vi "SVT Fractional-octave Analysis (1 Ch).vi"(0 "scaled signal [EU]":waveform(dbl)={"t0"=timestamp(0 s since 1904-01-01), "dt"=1.953125e-05, "Y"=[]}, 1 "restart averaging (F)":bool, 2 "reset filter (F)":bool, 5 "frequency range [Hz]":T9={"low frequency"=125.0, "high frequency"=8000.0} {"high frequency" min=0.001 format="%.2f"; "low frequency" min=0.001 format="%.2f"}, 7 "bandwidth":T2(ring)=enum."1/12 octave", 9 "dB On (T)":bool=TRUE, 11 "error in (no error)":errorcluster, 12 "averaging type":T7(ring), 13 "exp avg settings":T1={" mode"=enum."Fast", "time constant [ms]"=125.0} {"time constant [ms]" format="%.2f"}, 14 "equal confidence level [dB]":dbl=125.0 format="%.2f") -> (3 "filter settled":bool, 4 "octave spectrum":T8 {"band power" format="%.2f"; "nominal frequencies [Hz]" format="%.2f"}, 6 "unit label":string, 8 "total band power":dbl format="%.2f", 10 "octave info":T3={"standard"=enum."ANSI S1.11", "bandwidth"=enum."1 octave", "low band"=0, "high band"=0, "weighting filter"=0, "dB reference"=0.0, "dB On"=FALSE, "unit label"="", "channel name"="", "description"="", "engineering units"=1, "custom label"="", "spectrum type"=enum."magnitude", "spectral density"=FALSE, "filters settled"=FALSE} {"engineering units" items=["custom..."=0, "V"=1, "A"=21, "C"=30, "pC"=31, "s"=32, "-"=29, "Pa"=2, "N"=20, "g"=3, "m/s^2"=4, "m/s"=5, "m"=6, "mm/s"=12, "mm"=13, "micron/s"=14, "micron"=15, "in/s^2"=7, "in/s"=8, "in"=9, "mil/s"=10, "mil"=11, "rad/s^2"=16, "rad/s"=17, "rad"=18, "deg/s^2"=26, "deg/s"=27, "deg"=28, "RPM"=22, "cycle/s^2"=23, "Hz"=24, "cycle"=25, "strain"=19]; "dB reference" format="%.2e"; "weighting filter" items=["Linear", "A-weighting", "B-weighting", "C-weighting", "ITU-R 468-4", "Dolby", "CCITT", "C-message", "Wb", "Wc", "Wd", "We", "Wf", "Wh", "Wj", "Wk", "Wm", "AES17 20 kHz lowpass", "AES17 40 kHz lowpass", "AES17 20 kHz highpass", "AES17 40 kHz highpass"]}, 15 "error out":errorcluster)   [LabVIEW 2017, in "SoundVib_Octave.lvlib"]
doc: "LabVIEW no longer supports this VI. The SVT Fractional-octave Analysis VI is available for compatibility with previous versions of the LabVIEW Sound and Vibration Toolkit. This version of the SVT Fractional-octave Analysis VI performs a fractional-octave analysis on <B>scaled signal [EU]</B> in accordance with the IEC 1260 standard. This standard has been superseded by the new IEC 61260 standard. If you want to ensure compliance with the latter standard, use the SVT Fractional-octave Analysis VI, located on the Octave Analysis palette instead. You can use this polymorphic VI to perform fractional-octave analysis on a single channel or on N channels. The data type you wire to the <B>scaled signal [EU]</B> input determines the polymorphic instance to use."
uses:
  <vilib>/addons/Sound and Vibration/svt_Octave/SoundVib_Octave.lvlib
  <vilib>/addons/_NISVFA/_Shared subVIs/Controls/svc_Octave Info.ctl
  <vilib>/addons/_NISVFA/_Shared subVIs/Controls/svc_Octave Standard.ctl
  <vilib>/addons/_NISVFA/_Shared subVIs/Controls/svc_Weighting Filter Text Ring.ctl
  <vilib>/addons/_NISVFA/_Shared subVIs/Controls/svc_Engineering Units Text Ring.ctl
  <vilib>/addons/Sound and Vibration/svt_Octave_2014 standard/SoundVib_Octave_2014 standard.lvlib
panel:
  out "# samples to settle":u64
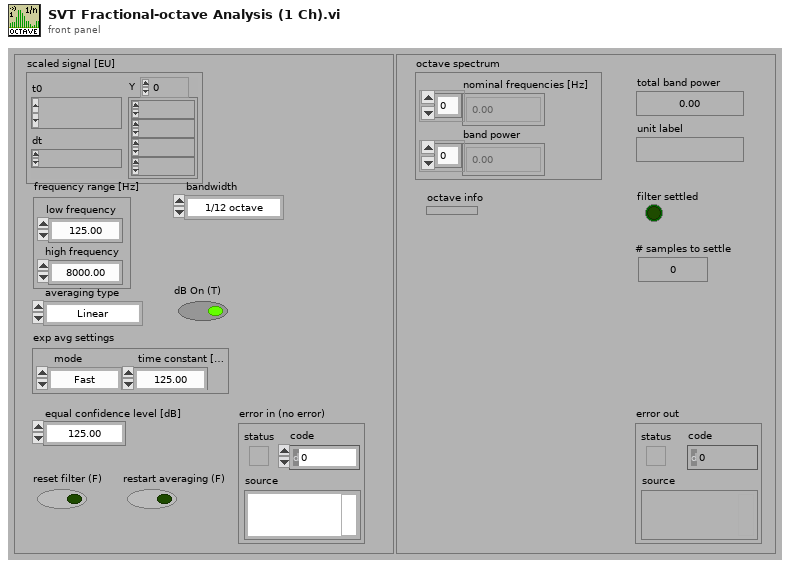
[diagram p1: front panel]
types:
  T1 = cluster{" mode":enum16{"Slow", "Fast", "Impulse", "Custom"}, "time constant [ms]":dbl}
  T2 = enum16{"1 octave", "1/3 octave", "1/6 octave", "1/12 octave", "1/24 octave"}
  T3 = typedef "svc_Octave Info.ctl" = cluster{"standard":T4, "bandwidth":enum16{"1 octave", "1/3 octave", "1/6 octave", "1/12 octave", "1/24 octave"}, "low band":i32, "high band":i32, "weighting filter":T5, "dB reference":dbl, "dB On":bool, "unit label":string, "channel name":string, "description":string, "engineering units":T6, "custom label":string, "spectrum type":enum16{"power", "magnitude"}, "spectral density":bool, "filters settled":bool}
  T4 = typedef "svc_Octave Standard.ctl" = enum16{"ANSI S1.11", "IEC 61260"}
  T5 = typedef "svc_Weighting Filter Text Ring.ctl" = u16
  T6 = typedef "svc_Engineering Units Text Ring.ctl" = u16
  T7 = enum16{"Linear", "Exponential", "Equal confidence", "Peak"}
  T8 = cluster{"nominal frequencies [Hz]":dbl[], "band power":dbl[]}
  T9 = cluster{"low frequency":dbl, "high frequency":dbl}
  T10 = cluster{"standard":T4, "bandwidth":enum16{"1 octave", "1/3 octave", "1/6 octave", "1/12 octave", "1/24 octave"}}
  T11 = cluster{"nominal frequencies [Hz]":dbl[], "band power [EU^2 rms]":dbl[]}
  T12 = cluster{"nominal frequencies [Hz]":dbl[], "band power [dB EU]":dbl[]}
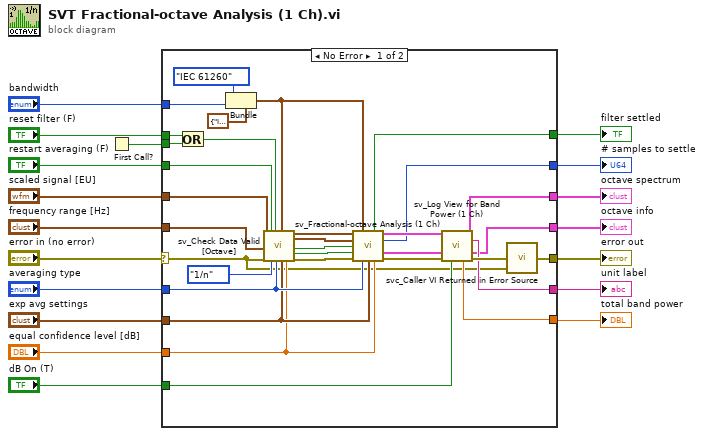
[diagram p0: block diagram]
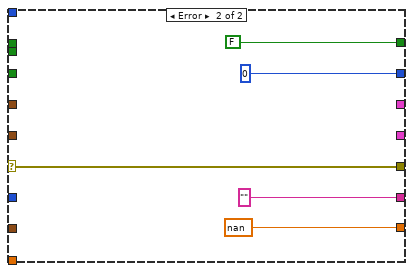
[diagram p2: hidden frame]
diagram:
  n1 = First Call?() -> (First Call?: T/F=w17:bool)
  n2 = case shown="No Error" "error in (no error)" {
    selector: "error in (no error)" -> [w21 w55]
    tunnel: w17 -> [w46 _]
    tunnel: [w45 nan ("total band power [dB EU]")] -> w16
    tunnel: [w24 FALSE ("settled?")] -> w15
    tunnel: "restart averaging (F)" -> [w44 _]
    tunnel: "averaging type" -> [w42 _]
    tunnel: "dB On (T)" -> [w41 _]
    tunnel: "frequency range [Hz]" -> [w39 _]
    tunnel: "bandwidth" -> [w30 _]
    tunnel: "exp avg settings" -> [w38 _]
    tunnel: "equal confidence level [dB]" -> [w25 _]
    tunnel: [w31 w55] -> w7
    tunnel: [w34 _] -> w6
    tunnel: [w33 "" ("unit label")] -> w5
    tunnel: [w32 _] -> w4
    tunnel: "scaled signal [EU]" -> [w29 _]
    tunnel: "reset filter (F)" -> [w47 _]
    tunnel: [w22 u64 0 ("# samples to settle")] -> w1
    frame No Error {
      n3 = Or(x=w47, y=w46) -> (x .or. y?=w26:bool)
      n4 = Bundle(cluster=T10 {"standard"=enum."IEC 61260", "bandwidth"=enum."1/3 octave"} ("1/n Octave settings"), "standard"=svc_Octave_Standard."IEC 61260", "bandwidth"=w30) -> (w27:T10)
      n5 = call <vilib>:"sv_Check Data Valid [Octave].vi"("scaled signal [EU]"=w29, "frequency range [Hz]"=w39, "error in (no error)"=w21, "restart averaging (F)"=w44, "bandwidth"=enum16{"1/1", "1/3", "1/n"}."1/n", "reset filter (F)"=w26, "averaging type"=w42, "1/n octave settings"=w27, "exp avg settings"=w38, "equal confidence level [dB]"=w25) -> ("dup scaled signal [EU]"=w49:waveform(dbl), "band number"=w37:cluster{"low band":i32, "high band":i32}, "Restart averaging"=w43:bool, "Reset Filter"=w28:bool, "error out"=w50:errorcluster)  [unwired: 5 in]
      n6 = call <vilib>:"sv_Fractional-octave Analysis (1 Ch).vi"("scaled signal [EU]"=w49, "1/n Octave settings"=w27, "band number"=w37, "restart averaging (F)"=w43, "reset filter (F)"=w28, "error in (no error)"=w50, "averaging type"=w42, "exp avg settings"=w38, "equal confidence level [dB]"=w25) -> ("settled?"=w24:bool, "octave spectrum"=w40:T11, "# samples to settle"=w22:u64, "octave info"=w35:T3, "error out"=w48:errorcluster)  [unwired: 2 in]
      n7 = call <vilib>:"sv_Log View for Band Power (1 Ch).vi"("octave spectrum"=w40, "octave info"=w35, "error in (no error)"=w48, "dB On (T)"=w41) -> ("octave spectrum"=w34:T12, "unit label"=w33:string, "octave info"=w32:T3, "total band power [dB EU]"=w45:dbl, "error out"=w36:errorcluster)  [unwired: 7 in]
      n8 = call <vilib>:"svc_Caller VI Returned in Error Source.vi"("warning input to caller"=w21, "error in (no error)"=w36) -> ("error out"=w31:errorcluster)  [unwired: 3 in]
    }
    frame Error {
    }
  }
  "filter settled" <- w15
  "unit label" <- w5
  "total band power" <- w16
  "error out" <- w7
  "octave spectrum" <- w6
  "octave info" <- w4
  "# samples to settle" <- w1
